vi "DUT Test 2.vi"(7 "DRV stand":T2, 8 "error in (no error)":errorcluster, 11 "DRV data":T1) -> (0 "error out":errorcluster, 2 "details":bool[](array[boolean]), 3 "DRV data 2":T1)   [LabVIEW 2018, in "Application.lvlib"]
uses:
  Application.lvlib
  DRV cluster 2.ctl
  DRV stand.ctl
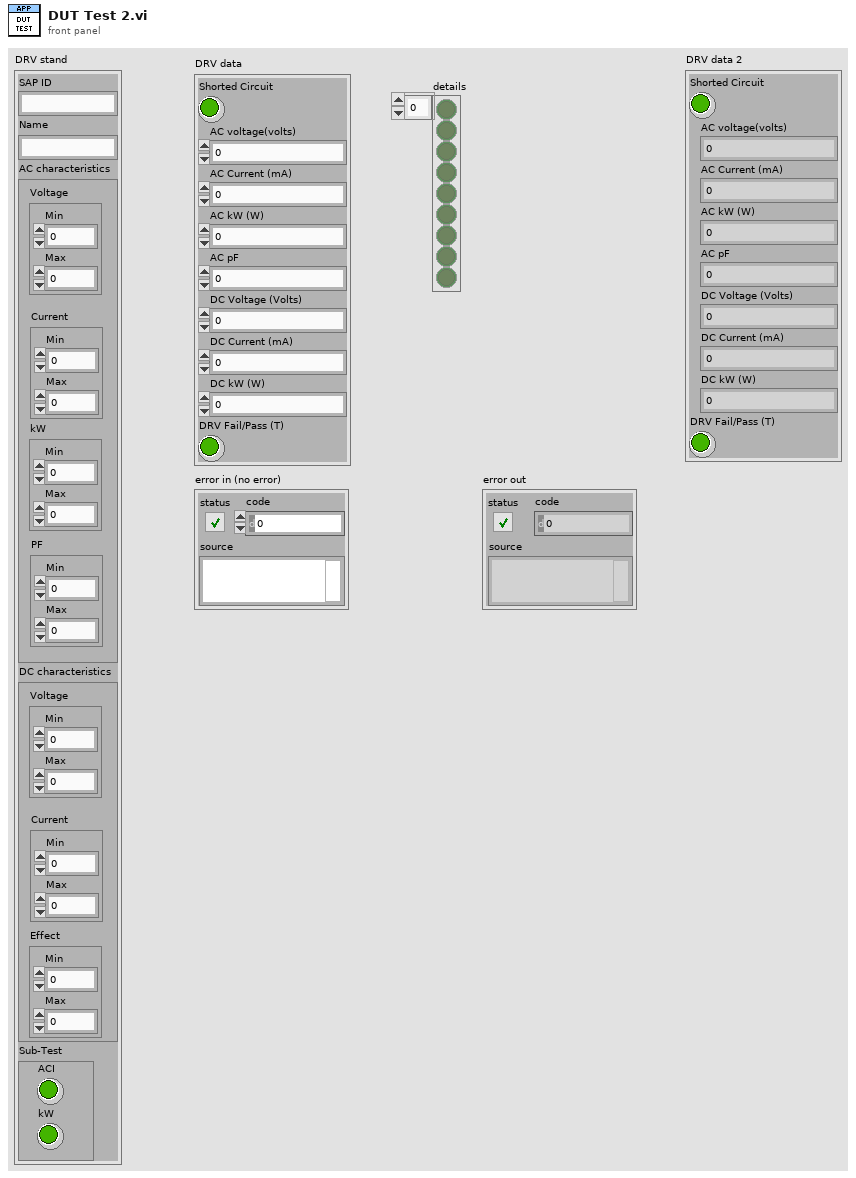
[diagram p1: front panel]
types:
  T1 = typedef "Application.lvlib/DRV cluster 2.ctl" = cluster{"Shorted Circuit":bool, "AC voltage(volts)":dbl, "AC Current (mA)":dbl, "AC kW (W)":dbl, "AC pF ":dbl, "DC Voltage (Volts)":dbl, "DC Current (mA)":dbl, "DC kW (W)":dbl, "DRV Fail/Pass (T)":bool}
  T2 = typedef "Application.lvlib/DRV stand.ctl" = cluster{"SAP ID":string, "Name":string, "AC characteristics":cluster{"Voltage":cluster{"Min":dbl, "Max":dbl}, "Current":cluster{"Min":dbl, "Max":dbl}, "kW":cluster{"Min":dbl, "Max":dbl}, "PF":cluster{"Min":dbl, "Max":dbl}}, "DC characteristics":cluster{"Voltage":cluster{"Min":dbl, "Max":dbl}, "Current":cluster{"Min":dbl, "Max":dbl}, "Effect":cluster{"Min":dbl, "Max":dbl}}, "Sub-Test":cluster{"ACV":bool, "ACI":bool, "kW":bool, "PF":bool, "DCV":bool, "DCI":bool, "efficiency":bool}}
  T3 = cluster{"ACV":bool, "ACI":bool, "kW":bool, "PF":bool, "DCV":bool, "DCI":bool, "efficiency":bool}
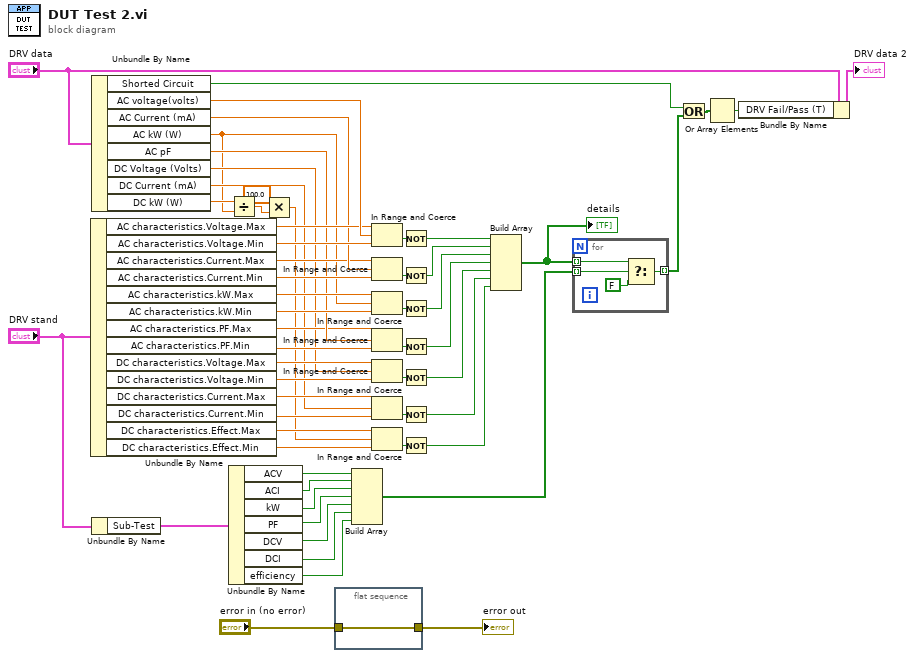
[diagram p0: block diagram]
diagram:
  n1 = Unbundle By Name("DRV stand") -> ("AC characteristics.Voltage.Max"=w49:dbl, "AC characteristics.Voltage.Min"=w48:dbl, "AC characteristics.Current.Max"=w46:dbl, "AC characteristics.Current.Min"=w45:dbl, "AC characteristics.kW.Max"=w44:dbl, "AC characteristics.kW.Min"=w43:dbl, "AC characteristics.PF.Max"=w41:dbl, "AC characteristics.PF.Min"=w40:dbl, "DC characteristics.Voltage.Max"=w39:dbl, "DC characteristics.Voltage.Min"=w38:dbl, "DC characteristics.Current.Max"=w36:dbl, "DC characteristics.Current.Min"=w35:dbl, "DC characteristics.Effect.Max"=w33:dbl, "DC characteristics.Effect.Min"=w32:dbl)
  n2 = Unbundle By Name("DRV data") -> ("Shorted Circuit"=w5:bool, "AC voltage(volts)"=w50:dbl, "AC Current (mA)"=w47:dbl, "AC kW (W)"=w26:dbl, "AC pF"=w42:dbl, "DC Voltage (Volts)"=w31:dbl, "DC Current (mA)"=w30:dbl, "DC kW (W)"=w27:dbl)
  n3 = Unbundle By Name("DRV stand") -> ("Sub-Test"=w14:T3)
  n4 = Divide(x=w27, y=w26) -> (x/y=w25:dbl)
  n5 = Unbundle By Name(w14) -> ("ACV"=w13:bool, "ACI"=w12:bool, "kW"=w11:bool, "PF"=w10:bool, "DCV"=w9:bool, "DCI"=w8:bool, "efficiency"=w7:bool)
  n6 = Multiply(x=100.0, y=w25) -> (x*y=w23:dbl)
  n7 = flat-sequence {
    tunnel: [w58] -> w54
    tunnel: "error in (no error)" -> [w58]
    frame #0 {
    }
  }
  n8 = Build Array(w13, w12, w11, w10, w9, w8, w7) -> (w3:bool[])
  n9 = In Range and Coerce(upper limit=w49, x=w50, lower limit=w48) -> (In Range?=w57:bool)  [unwired: 1 out]
  n10 = In Range and Coerce(upper limit=w46, x=w47, lower limit=w45) -> (In Range?=w51:bool)  [unwired: 1 out]
  n11 = In Range and Coerce(upper limit=w44, x=w26, lower limit=w43) -> (In Range?=w56:bool)  [unwired: 1 out]
  n12 = In Range and Coerce(upper limit=w41, x=w42, lower limit=w40) -> (In Range?=w55:bool)  [unwired: 1 out]
  n13 = In Range and Coerce(upper limit=w39, x=w31, lower limit=w38) -> (In Range?=w52:bool)  [unwired: 1 out]
  n14 = In Range and Coerce(upper limit=w36, x=w30, lower limit=w35) -> (In Range?=w37:bool)  [unwired: 1 out]
  n15 = In Range and Coerce(upper limit=w33, x=w23, lower limit=w32) -> (In Range?=w34:bool)  [unwired: 1 out]
  n16 = Not(x=w57) -> (.not. x?=w22:bool)
  n17 = Not(x=w51) -> (.not. x?=w21:bool)
  n18 = Not(x=w56) -> (.not. x?=w20:bool)
  n19 = Not(x=w55) -> (.not. x?=w19:bool)
  n20 = Not(x=w52) -> (.not. x?=w18:bool)
  n21 = Not(x=w37) -> (.not. x?=w17:bool)
  n22 = Not(x=w34) -> (.not. x?=w16:bool)
  n23 = Build Array(w22, w21, w20, w19, w18, w17, w16) -> (w1:bool[])
  "details" <- w1
  n24 = for {
    tunnel: w3 -> [w62] mode=indexing
    tunnel: w1 -> [w61] mode=indexing
    tunnel: [w59] -> w2 mode=indexing
    n25 = Select(t=w61, s=w62, f=FALSE) -> (s? t:f=w59:bool)
  }
  n26 = Or(x=w5, y=w2) -> (x .or. y?=w4:bool[])
  n27 = Or Array Elements(Boolean array=w4) -> (logical OR=w6:bool)
  n28 = Bundle By Name(cluster="DRV data", "DRV Fail/Pass (T)"=w6) -> (→"DRV data 2":T1)
  "error out" <- w54
